vi "COM Port Select.vi"(8 "error in (no error)":errorcluster, 10 "T Button Name (\"OK\")":string="OK") -> (0 "error out":errorcluster, 3 "OK":bool)   [LabVIEW 2018]
uses:
  CTL/FGV - R-W.ctl
panel:
  in  "COM PORT":refnum<visa-resource-name>="COM3"
  in  "OK":bool
  out "Display Message":string caption="Message"
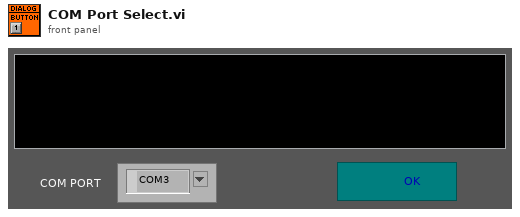
[diagram p1: front panel]
types:
  T1 = typedef "FGV - R-W.ctl" = enum16{"W", "R"}
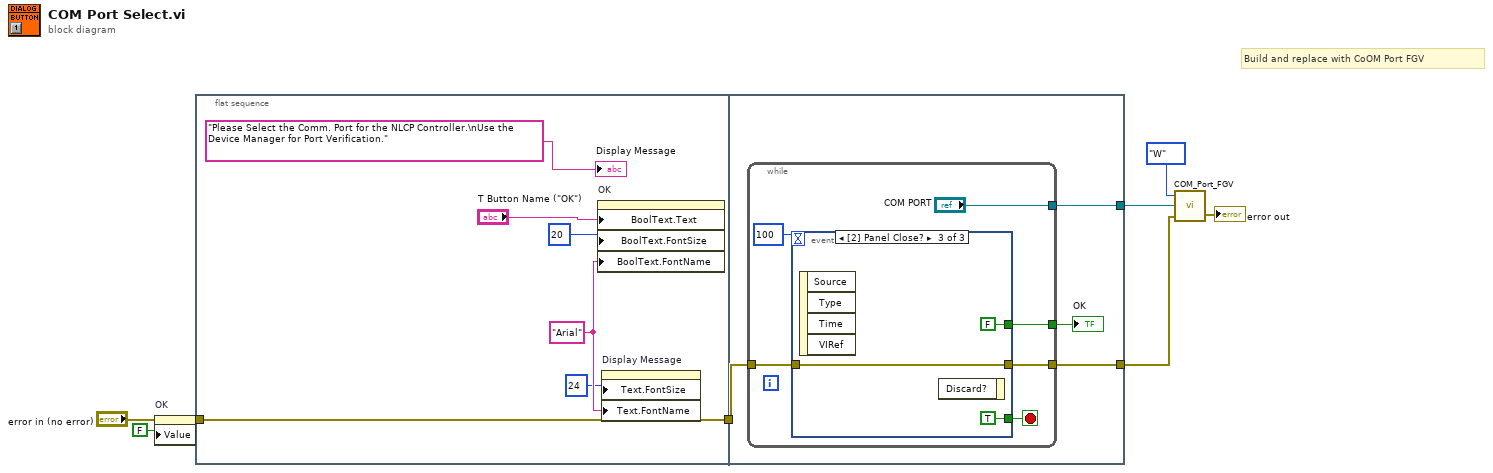
[diagram p0: block diagram]
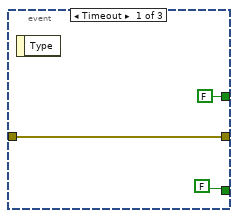
[diagram p2: hidden frame]
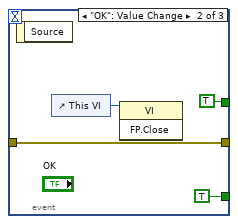
[diagram p3: hidden frame]
diagram:
  # "Build and replace with CoOM Port FGV"
  n1 = property on="OK" class="Bool (strict)"(error in="error in (no error)", "Value"=FALSE ("OK")) -> (error out=w6:errorcluster)  [unwired: 1 in, 1 out]
  n2 = flat-sequence {
    tunnel: [w9] -> w8
    tunnel: w6 -> [w9]
    tunnel: w8 -> [w18]
    tunnel: [w17] -> w2
    tunnel: [w16] -> w4
    frame #0 {
      w12 = "Arial" ("Font Name")
      n3 = property on="OK" class="Bool"("BoolText.Text"="T Button Name (\"OK\")", "BoolText.FontSize"=u32 20 ("Boolean Text.Font:Size"), "BoolText.FontName"=w12) -> ()  [unwired: 2 in, 2 out]
      n4 = property on="Display Message" class="Str"("Text.FontSize"=u32 24 ("Text.Font:Size"), "Text.FontName"=w12) -> ()  [unwired: 2 in, 2 out]
      "Display Message" <- "Please Select the Comm. Port for the NLCP Controller.\nUse the Device Manager for Port Verification." ("message")
    }
    frame #1 {
      n5 = while {
        tunnel: [w22] -> w15
        tunnel: w18 -> [w20]
        tunnel: [w21] -> w17
        tunnel: ["COM PORT"] -> w16
        stop <- w23 stop-if-true
        n6 = event shown="[2] Panel Close?" {
          selector: _ -> [_ _ _]
          dyn-events: _ -> [_ _ _]
          timeout: 100 -> [_ _ _]
          tunnel: [FALSE TRUE TRUE] -> w23
          tunnel: [FALSE TRUE FALSE] -> w22
          tunnel: [w25 w29 w32] -> w21
          tunnel: w20 -> [w25 w29 w32]
          event Timeout {
            n7 = event-data() -> ()  [unwired: 2 out]
          }
          event "OK": Value Change {
            n8 = event-data() -> ()  [unwired: 2 out]
            n9 = control-ref of="This VI"() -> (w28:refnum<vi>)
            n10 = invoke class="VI" method="FP.Close"(reference=w28) -> ()  [unwired: 2 in, 3 out]
          }
          event Panel Close? {
            n11 = event-data() -> ()  [unwired: 5 out]
            n12 = event-data() -> ()  [unwired: 2 in, 1 out]
          }
        }
      }
      "OK" <- w15
    }
  }
  n13 = call "COM_Port_FGV.vi"("error in (no error)"=w2, "COM Port In"=w4, "Action"=FGV_-_R-W."W") -> ("error out"=→"error out":errorcluster)  [unwired: 1 out]
